vi "SR830-3_Open_Queue.vi"(8 "error in (no error)":errorcluster) -> (0 "error out":errorcluster, 2 "queue out":refnum<queue>)   [LabVIEW 2018]
uses:
  SR830/SR830-Cluster.ctl
  Global/Global Variables/Queues_global.vi
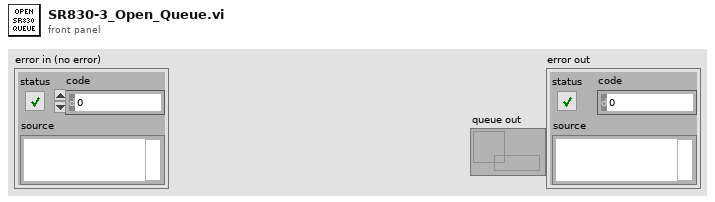
[diagram p1: front panel]
types:
  T1 = typedef "SR830-Cluster.ctl" = cluster{"Lockin 1":dbl[][], "X1-Display":dbl, "Y1-Display":dbl, "X1 Percent":dbl, "X1 Overload":bool, "Y1 Overload":bool, "Unit X1":string, "Unit X2":string, "Unit X2a":string, "Unit X1a":string, "Sensitivity Setpoint":i16, "X1 Percent 2":dbl, "Y1":dbl, "X1":dbl, "Preamp OVL":bool}
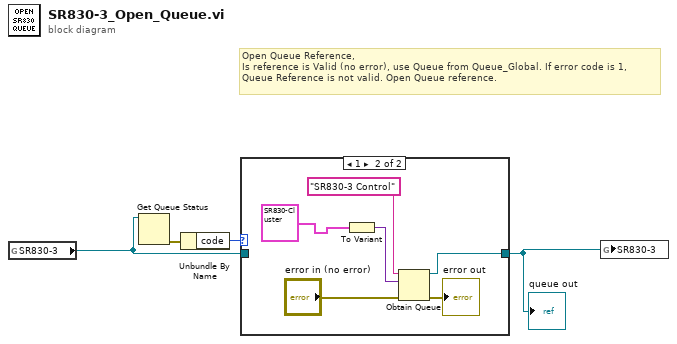
[diagram p0: block diagram]
diagram:
  # "Open Queue Reference, \nIs reference is Valid (no error), use Queue from Queue_Global. If error code is 1, \nQueue Reference is not valid. Open Queue reference."
  n1 = global read "Queues_global.vi" "SR830-3"() -> (w2:refnum<queue>)
  n2 = Get Queue Status(queue=w2) -> (error out=w4:errorcluster)  [unwired: 2 in, 7 out]
  n3 = Unbundle By Name(w4) -> ("code"=w3:i32)
  n4 = case shown="1" w3 {
    tunnel: [w5 w7] -> w1
    tunnel: w2 -> [w5 _]
    frame 0, Default {
    }
    frame 1 {
      n5 = To Variant(anything=T1 {"Lockin 1"=[], "X1-Display"=0.0, "Y1-Display"=0.0, "X1 Percent"=0.0, "X1 Overload"=FALSE, "Y1 Overload"=FALSE, "Unit X1"="nV", "Unit X2"="nV", "Unit X2a"="nV", "Unit X1a"="nV", "Sensitivity Setpoint"=26, "X1 Percent 2"=0.0, "Y1"=0.0, "X1"=0.0, "Preamp OVL"=FALSE} ("SR830")) -> (Variant=w10:variant)
      n6 = Obtain Queue(name (unnamed)="SR830-3 Control", element data type=w10, error in (no error)="error in (no error)") -> (queue out=w7:refnum<queue>, error out=→"error out":errorcluster)  [unwired: 2 in, 1 out]
    }
  }
  "queue out" <- w1
  n7 = global write "Queues_global.vi" "SR830-3"(w1) -> ()
